vi "Read Device Information.vi"(8 "error in (no error)":errorcluster, 11 "PLBB in":refnum<class "PL BlackBox Modbus Client.lvclass">) -> (0 "error out":errorcluster, 2 "device information":T1, 3 "PLBB out":refnum<class "PL BlackBox Modbus Client.lvclass">)   [LabVIEW 2015, in "PL BlackBox Modbus Client.lvclass"]
doc: "Reads the device information."
uses:
  PL BlackBox Modbus Client.lvclass
  <vilib>/plasmapper/PL Modbus Client/PL Modbus Client.lvclass
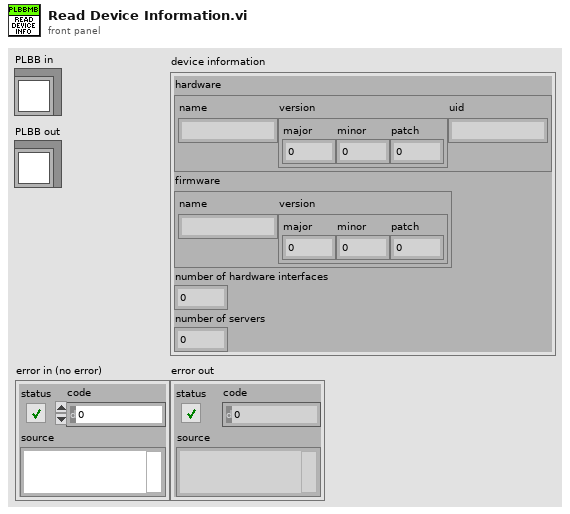
[diagram p1: front panel]
types:
  T1 = cluster{"hardware":cluster{"name":string, "version":cluster{"major":u16, "minor":u16, "patch":u16}, "uid":string}, "firmware":cluster{"name":string, "version":cluster{"major":u16, "minor":u16, "patch":u16}}, "number of hardware interfaces":u16, "number of servers":u16}
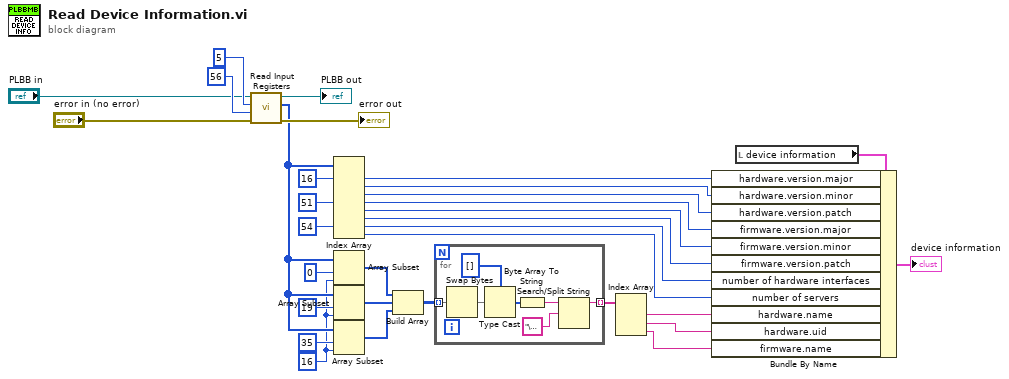
[diagram p0: block diagram]
diagram:
  w7 = 16 ("index")
  n1 = call <vilib>:"Read Input Registers.vi"("error in (no error)"="error in (no error)", "number of input registers"=u16 56 ("address"), "address"=u16 5, "MODBUS in"="PLBB in") -> ("error out"=→"error out":errorcluster, "values"=w8:u16[], "MODBUS out"=→"PLBB out":refnum<class "PL BlackBox Modbus Client.lvclass">)  [unwired: 5 in]
  n2 = Index Array(array=w8, index #1=16 ("index"), index #4=51 ("index"), index #7=54 ("index")) -> (element #1=w24:u16, element #2=w23:u16, element #3=w22:u16, element #4=w21:u16, element #5=w20:u16, element #6=w19:u16, element #7=w18:u16, element #8=w17:u16)  [unwired: 5 in]
  n3 = Array Subset(array=w8, index=0, length=w7) -> (w6:u16[])
  n4 = Array Subset(array=w8, index=19, length=w7) -> (w5:u16[])
  n5 = Array Subset(array=w8, index=35, length=w7) -> (w4:u16[])
  n6 = Build Array(w6, w5, w4) -> (w3:u16[][])
  n7 = for {
    tunnel: [w34] -> w15 mode=indexing
    tunnel: w3 -> [w33] mode=indexing
    n8 = Swap Bytes(anything=w33) -> (byte swapped=w37:u16[])
    n9 = Type Cast(type=u8[] [] ("values"), x=w37) -> (*(type *) &x=w39:u8[])
    n10 = Byte Array To String(unsigned byte array=w39) -> (string=w36:string)
    n11 = Search/Split String(string=w36, search string/char (-)="\u0000") -> (substring before match=w34:string)  [unwired: 1 in, 2 out]
  }
  n12 = Index Array(array=w15) -> (element #1=w14:string, element #2=w13:string, element #3=w12:string)  [unwired: 3 in]
  n13 = local read "device information"() -> (w25:T1)
  n14 = Bundle By Name(cluster=w25, "hardware.version.major"=w24, "hardware.version.minor"=w23, "hardware.version.patch"=w22, "firmware.version.major"=w21, "firmware.version.minor"=w20, "firmware.version.patch"=w19, "number of hardware interfaces"=w18, "number of servers"=w17, "hardware.name"=w14, "hardware.uid"=w13, "firmware.name"=w12) -> (→"device information":T1)
